vi "Save Text.vi"(8 "error in (no error)":errorcluster, 10 "Data":dbl, 11 "CSV in":refnum<class "CSV.lvclass">) -> (0 "error out":errorcluster, 3 "Text File out":refnum<class "Text File.lvclass">)   [LabVIEW 2020, in "Text File.lvlib" / "CSV.lvlib" / "CSV.lvclass"]
uses:
  CSV.lvclass
  C:/Users/Asus/Dropbox/trabajos_apuntes/7 semestre/labview/Actor Framework Tarea/Text File/Text File/Text File.lvclass
  Text File/Text File/Text File.lvclass
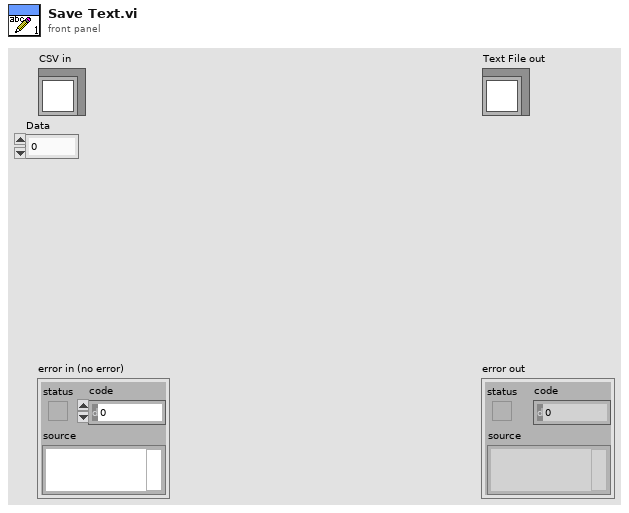
[diagram p1: front panel]
types:
  T1 = enum16{"open", "replace", "create", "open or create", "replace or create", "replace or create with confirmation"}
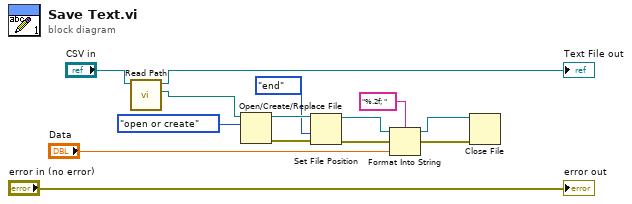
[diagram p0: block diagram]
diagram:
  n1 = call-dynamic "Read Path.vi"("Text File in"="CSV in") -> ("Path"=w3:path, "Text File out"=→"Text File out":refnum<class "CSV.lvclass">)  [unwired: 8 in, 1 out]
  n2 = Open/Create/Replace File(file path (use dialog)=w3, operation (0:open)=T1."open or create") -> (refnum out=w12:refnum<file>, error out=w13:errorcluster)  [unwired: 4 in, 1 out]
  n3 = Set File Position(refnum=w12, from (0:start)=enum16{"start", "end", "current"}."end", error in=w13) -> (refnum out=w9:refnum<file>, error out=w10:errorcluster)  [unwired: 1 in]
  n4 = Format Into String(format string="%.2f; ", initial string=w9, error in=w10, "Data") -> (resulting string=w7:refnum<file>, error out=w8:errorcluster)
  n5 = Close File(refnum=w7, error in=w8) -> ()  [unwired: 2 out]
  "error out" <- "error in (no error)"
